vi "proc_timeout.vi"(4 "error in":errorcluster, 6 "vars runtime":T2, 7 "vars general":T1) -> (0 "error out":errorcluster, 2 "vars runtime":T2, 3 "vars general":T1)   [LabVIEW 2015]
uses:
  Type Definitions/vars_runtime.ctl
  Type Definitions/vars_settings.ctl
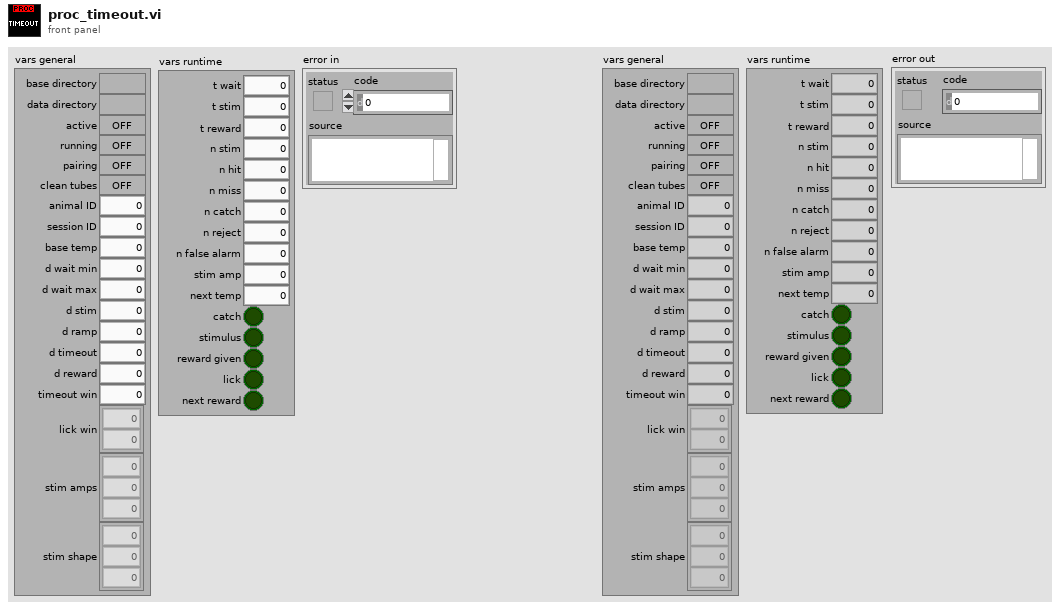
[diagram p1: front panel]
types:
  T1 = typedef "vars_settings.ctl" = cluster{"base directory":path, "data directory":path, "active":bool, "running":bool, "pairing":bool, "clean tubes":bool, "animal ID":u16, "session ID":u16, "base temp":sgl, "d wait min":u16, "d wait max":u16, "d stim":u16, "d ramp":u16, "d timeout":u16, "d reward":u16, "timeout win":u16, "lick win":i32[], "stim amps":dbl[], "stim shape":dbl[]}
  T2 = typedef "vars_runtime.ctl" = cluster{"t wait":u16, "t stim":u16, "t reward":u16, "n stim":u16, "n hit":u16, "n miss":u16, "n catch":u16, "n reject":u16, "n false alarm":u16, "stim amp":sgl, "next temp":sgl, "catch":bool, "stimulus":bool, "reward given":bool, "lick":bool, "next reward":bool}
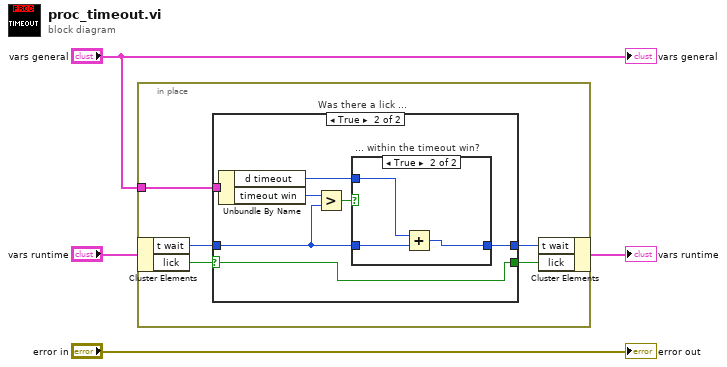
[diagram p0: block diagram]
diagram:
  n1 = in-place {
    in-place-border: "vars general" -> [w7]
    n2 = in-place-cluster #1("vars runtime") -> ("t wait"=w9:u16, "lick"=w6:bool)
    n3 = case "Was there a lick ..." shown="True" w6 {
      selector: w6 -> [w11 w16]
      tunnel: w9 -> [w10 w13]
      tunnel: [w10 w17] -> w8
      tunnel: w7 -> [_ w18]
      tunnel: [w11 w16] -> w5
      frame False {
        # "Continue waiting (decrement wait counter)"
      }
      frame True {
        # "Initialize stimulus; get new waiting time"
        n4 = Unbundle By Name(w18) -> ("d timeout"=w12:u16, "timeout win"=w14:u16)
        n5 = Greater?(x=w14, y=w13) -> (0:w15:bool)
        n6 = case "... within the timeout win?" shown="True" w15 {
          tunnel: [w19 w22] -> w17
          tunnel: w13 -> [w19 w21]
          tunnel: w12 -> [_ w20]
          frame False {
          }
          frame True {
            n7 = Add(x=w20, y=w21) -> (x+y=w22:u16)
          }
        }
      }
    }
    n8 = in-place-cluster #1("t wait"=w8, "lick"=w5) -> (→"vars runtime":T2)
  }
  "vars general" <- "vars general"
  "error out" <- "error in"
